vi "Destroy.vi"(0 "LibWriter":refnum<class "LibWriter.lvclass">, 5 "error in (no error)":errorcluster) -> (19 "error out":errorcluster)   [LabVIEW 2014, in "LibWriter.lvclass"]
doc: "Destroys an object created with a ClassWriter constructor VI or a subclass of the ClassWriter class. This VI must be reentrant.\n\n[GOOP 2.0.16]"
uses:
  <resource>/Framework/Providers/Open_GDS/ClassProviders/LibProvider_BaseClassInterface/LibWriter_class/ClassWriter_class/LibWriter.lvclass
  <resource>/Framework/Providers/Open_GDS/ClassProviders/LibProvider_BaseClassInterface/LibWriter_class/ClassWriter_class/LibWriter.lvclass/LibWriter.ctl
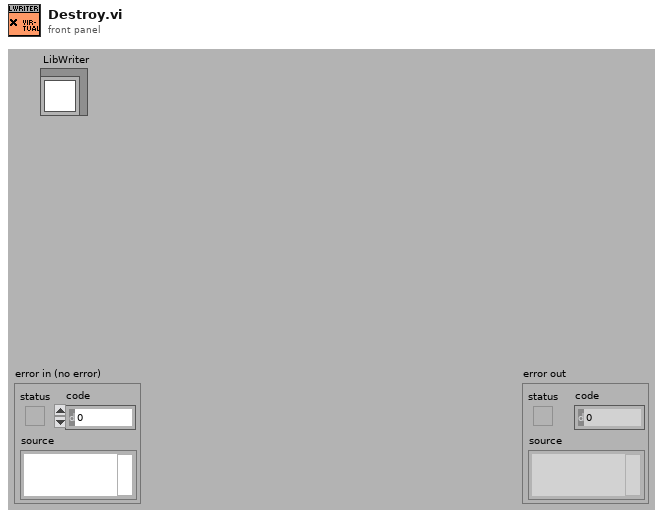
[diagram p1: front panel]
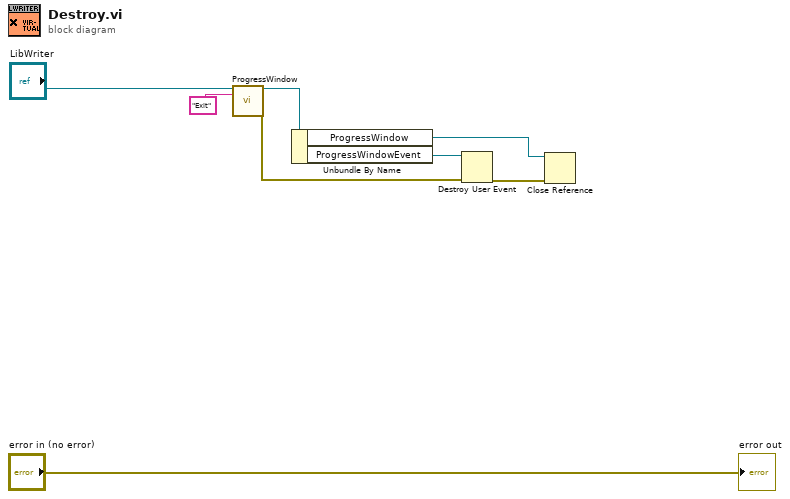
[diagram p0: block diagram]
diagram:
  n1 = call-dynamic "ProgressWindow.vi"("LibWriter"="LibWriter", "Message(Exit)"="Exit") -> ("LibWriter"=w5:refnum<class "LibWriter.lvclass">, "error out"=w3:errorcluster)  [unwired: 16 in]
  n2 = Unbundle By Name(w5) -> ("ProgressWindow"=w1:refnum<vi>, "ProgressWindowEvent"=w4:refnum<user-event>)
  n3 = Destroy User Event(user event=w4, error in=w3) -> (error out=w2:errorcluster)
  n4 = Close Reference(reference=w1, error in (no error)=w2) -> ()  [unwired: 1 out]
  "error out" <- "error in (no error)"
